vi "RSZVB Set ALC Port Clamp.vi"(7 "Clamp State (Off)":bool, 8 "error in (no error)":errorcluster {"code" format="%.0x"}, 9 "Port (1)":i32=1, 10 "Channel (1)":i32=1, 11 "VISA session":refnum<visa-resource-name>) -> (0 "error out":errorcluster {"code" format="%.0x"}, 3 "dup VISA session":refnum<visa-resource-name>)   [LabVIEW 2011]
doc: "Suspends the ALC mechanism at source port <Pt> while the analyzer acquires measurement data (Clamp ALC during Measurement). \n\nRemote-control command(s):\nSOURce<Ch>:POWer<Pt>:ALC:CLAMp"
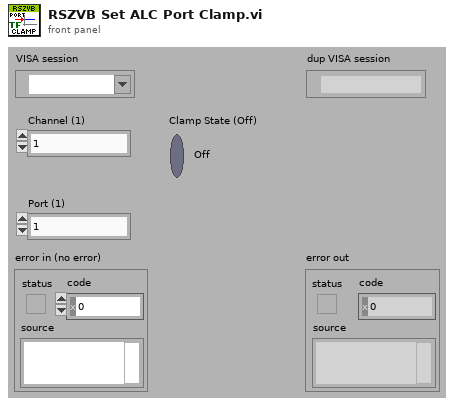
[diagram p1: front panel]
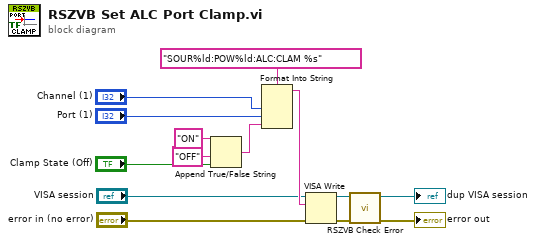
[diagram p0: block diagram]
diagram:
  n1 = Append True/False String(1:"Clamp State (Off)", 2:"OFF" ("false string"), 3:"ON" ("true string")) -> (0:w11:string)  [unwired: 1 in]
  n2 = Format Into String(format string="SOUR%ld:POW%ld:ALC:CLAM %s", "Channel (1)", "Port (1)", w11) -> (resulting string=w10:string)  [unwired: 2 in, 1 out]
  n3 = VISA Write(VISA resource name="VISA session", write buffer=w10, error in (no error)="error in (no error)") -> (VISA resource name out=w8:refnum<visa-resource-name>, error out=w9:errorcluster)  [unwired: 1 out]
  n4 = call "RSZVB Check Error.vi"("error in (no error)"=w9, "VISA session"=w8) -> ("error out"=→"error out":errorcluster, "dup VISA session"=→"dup VISA session":refnum<visa-resource-name>)  [unwired: 8 in]
